vi "ChassisRefSelector.vi"(11 "Enum 2":T1) -> (3 "String":string)   [LabVIEW 2014, in "ChassisLib.lvlib"]
uses:
  ChassisLib.lvlib
  ChassisRefs.ctl
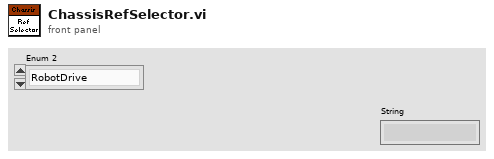
[diagram p1: front panel]
types:
  T1 = typedef "ChassisLib.lvlib/ChassisRefs.ctl" = enum16{"RobotDrive", "Compressor", "DriveEncoderLeft", "DriveEncoderRight"}
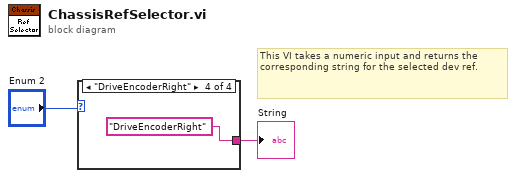
[diagram p0: block diagram]
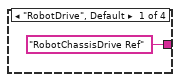
[diagram p2: hidden frame]
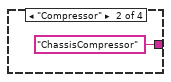
[diagram p3: hidden frame]
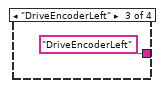
[diagram p4: hidden frame]
diagram:
  # "This VI takes a numeric input and returns the corresponding string for the selected dev ref."
  n1 = case shown="\"DriveEncoderRight\"" "Enum 2" {
    tunnel: ["RobotChassisDrive Ref" "ChassisCompressor" "DriveEncoderLeft" "DriveEncoderRight"] -> w2
    frame "RobotDrive", Default {
    }
    frame "Compressor" {
    }
    frame "DriveEncoderLeft" {
    }
    frame "DriveEncoderRight" {
    }
  }
  "String" <- w2
